vi "protocoljunk.vi"() -> ()   [LabVIEW 2013]
panel:
  out "hex integer string":string[](array[string])
  out "error out":errorcluster
  in  "error in":errorcluster
  out "index":i32
  out "Hex String":string
  out "Value in Flpating Point":dbl
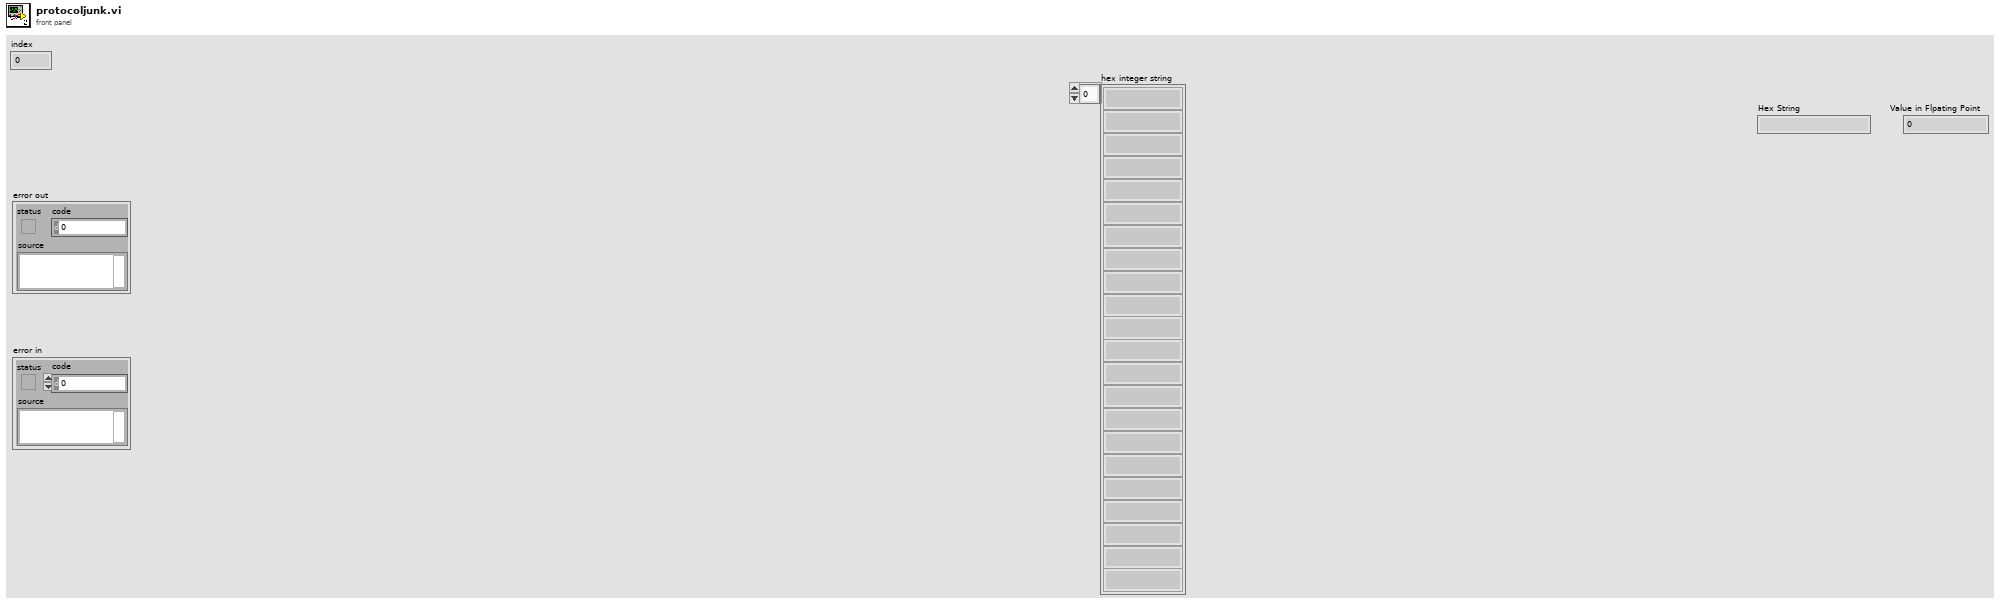
[diagram p1: front panel]
types:
  T1 = enum16{"big-endian, network order", "native, host order", "little-endian"}
  T2 = enum16{"open", "replace", "create", "open or create", "replace or create", "replace or create with confirmation"}
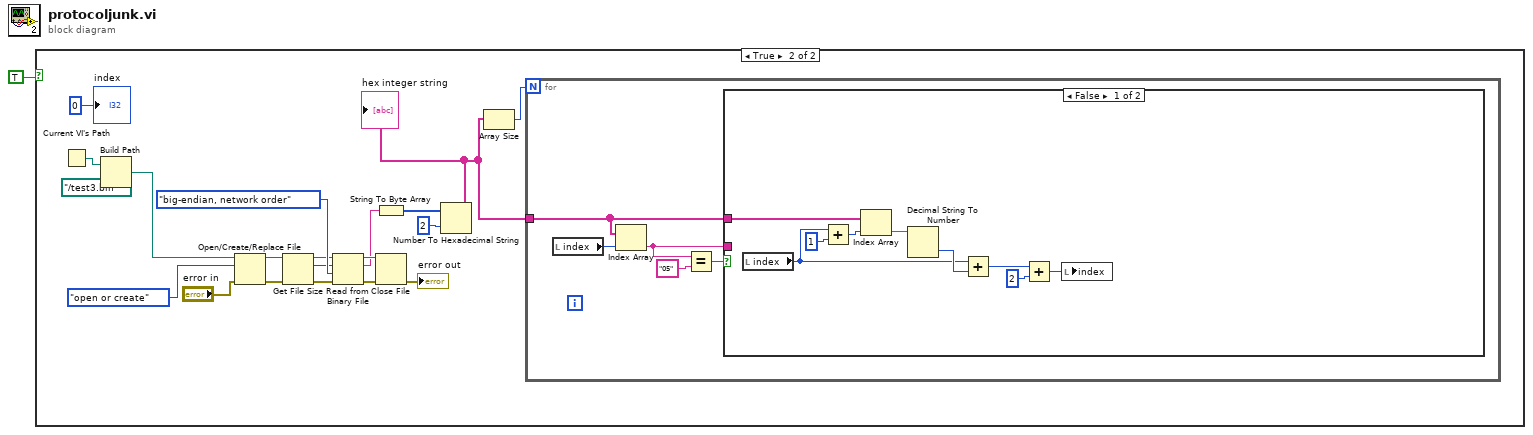
[diagram p0: block diagram]
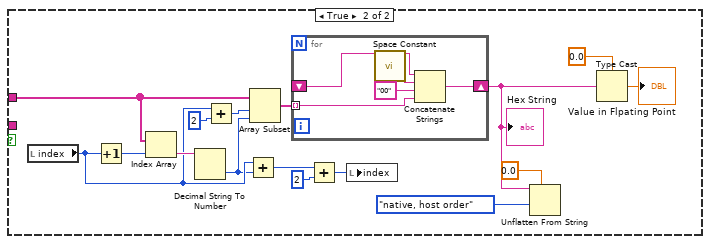
[diagram p3: hidden frame]
diagram:
  n1 = case shown="True" TRUE {
    frame False {
    }
    frame True {
      n2 = Current VI's Path() -> (path=w4:path)
      n3 = Build Path(base path=w4, name or relative path=path "../test3.bin") -> (appended path=w3:path)
      n4 = Open/Create/Replace File(file path (use dialog)=w3, error in="error in", operation (0:open)=T2."open or create") -> (refnum out=w15:refnum<file>, error out=w13:errorcluster)  [unwired: 3 in, 1 out]
      n5 = Get File Size(file=w15, error in=w13) -> (refnum out=w14:refnum<file>, size (in bytes)=w11:i64, 0:w12:errorcluster)
      n6 = Read from Binary File(8:w12, 9:T1."big-endian, network order" ("byte order (0:big-endian, network order)"), 10:w11, 11:w14) -> (0:w18:errorcluster, 2:w10:string, 3:w16:refnum<file>)  [unwired: 2 in, 1 out]
      n7 = String To Byte Array(string=w10) -> (unsigned byte array=w9:u8[])
      n8 = Close File(refnum=w16, error in=w18) -> (error out=→"error out":errorcluster)  [unwired: 1 out]
      n9 = Number To Hexadecimal String(1:2, 2:w9) -> (0:w7:string[])
      "hex integer string" <- w7
      n10 = Array Size(array=w7) -> (size(s)=w5:i32)
      n11 = for {
        N: w5 -> [_]
        tunnel: w7 -> [w24]
        n12 = local read "index"() -> (w22:i32)
        n13 = Index Array(array=w24, index=w22) -> (element=w23:string)
        n14 = Equal?(x=w23, y="05") -> (x = y?=w25:bool)
        n15 = case shown="False" w25 {
          tunnel: w24 -> [w33 w48]
          tunnel: w23 -> [_ _]
          frame False {
            n16 = local read "index"() -> (w30:i32)
            n17 = Add(x=w30, y=1) -> (x+y=w31:i32)
            n18 = Index Array(array=w33, index=w31) -> (element=w35:string)
            n19 = Decimal String To Number(string=w35) -> (number=w34:i32)  [unwired: 2 in, 1 out]
            n20 = Add(x=w30, y=w34) -> (x+y=w29:i32)
            n21 = Add(x=w29, y=2) -> (x+y=w27:i32)
            n22 = local write "index"(w27) -> ()
          }
          frame True {
            n23 = local read "index"() -> (w46:i32)
            n24 = Increment(x=w46) -> (x+1=w51:i32)
            n25 = Index Array(array=w48, index=w51) -> (element=w49:string)
            n26 = Decimal String To Number(string=w49) -> (number=w42:i32)  [unwired: 2 in, 1 out]
            n27 = Add(x=w46, y=2) -> (x+y=w44:i32)
            n28 = Add(x=w46, y=w42) -> (x+y=w47:i32)
            n29 = Array Subset(array=w48, index=w44, length=w42) -> (w41:string[])
            n30 = for {
              tunnel: w41 -> [w55] mode=indexing
              shift-right: [w56] -> w36
              shift-left: _ -> [w54]
              n31 = call <vilib>:"Space Constant.vi"() -> ("String"=w52:string)
              n32 = Concatenate Strings(w54, w52, "00", w55) -> (w56:string)
            }
            "Hex String" <- w36
            n33 = Add(x=w47, y=2) -> (x+y=w43:i32)
            n34 = local write "index"(w43) -> ()
            n35 = Unflatten From String(type=0.0, binary string=w36, byte order (0:big-endian, network order)=T1."native, host order") -> ()  [unwired: 2 in, 3 out]
            n36 = Type Cast(type=0.0, x=w36) -> (*(type *) &x=→"Value in Flpating Point":dbl)
          }
        }
      }
      "index" <- 0
    }
  }
